vi "Frame Data FGV [Color].vi"(6 "Command":enum16{"Get", "Initialize"}(ring), 8 "error in (no error)":errorcluster, 10 "FrameDescription":T1) -> (0 "error out":errorcluster, 2 "Byte Array":u8[](array[numeric]))   [LabVIEW 2011, in "LVH-KinectOne.lvlib"]
uses:
  LVH-KinectOne.lvlib
  Type Defs/FrameDescription.ctl
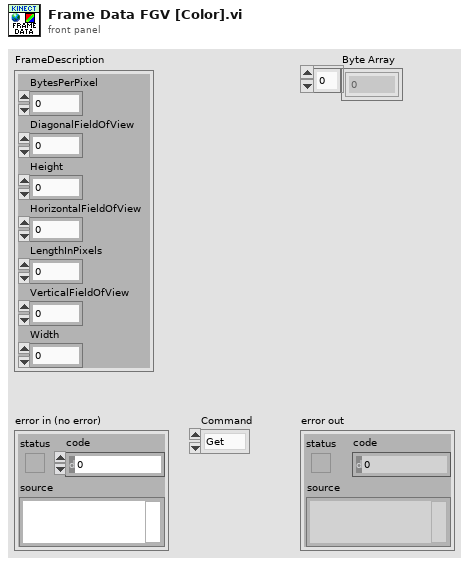
[diagram p1: front panel]
types:
  T1 = typedef "LVH-KinectOne.lvlib/FrameDescription.ctl" = cluster{"BytesPerPixel":u32, "DiagonalFieldOfView":sgl, "Height":i32, "HorizontalFieldOfView":sgl, "LengthInPixels":u32, "VerticalFieldOfView":sgl, "Width":i32}
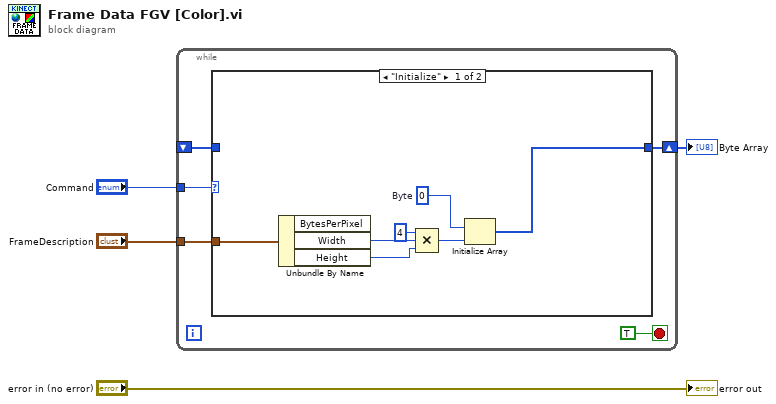
[diagram p0: block diagram]
diagram:
  n1 = while {
    tunnel: "Command" -> [w9]
    tunnel: "FrameDescription" -> [w8]
    shift-right: [w7] -> w2
    shift-left: _ -> [w6]
    stop <- TRUE stop-if-true
    n2 = case shown="\"Initialize\"" w9 {
      tunnel: w8 -> [w14 _]
      tunnel: [w11 w17] -> w7
      tunnel: w6 -> [_ w17]
      frame "Initialize" {
        w15 = u8 0  # Byte
        n3 = Unbundle By Name(w14) -> ("Width"=w13:i32, "Height"=w12:i32)  [unwired: 1 out]
        n4 = Compound Arithmetic op=MULTIPLY(4 ("value"), w13, w12) -> (w16:i32)
        n5 = Initialize Array(w15, w16) -> (w11:u8[])
      }
      frame "Get", Default {
      }
    }
  }
  "Byte Array" <- w2
  "error out" <- "error in (no error)"
